vi "Execute Command Script.vi"(7 "Micropulse # In":i32, 8 "error in (no error)":errorcluster, 10 "String in":string) -> (0 "error out":errorcluster, 2 "Transmitted string out":string, 5 "Micropulse # Out":i32)   [LabVIEW 2026, in "MicroPulse_Driver.lvlib"]
doc: "Execute a native Micropulse command (or set of commands separated by carriage returns).\n\n<b>IMPORTANT:</b> Only use this VI if you are familiar with the Micropulse command set and are confident that the commands you are entering are free from errors."
uses:
  MicroPulse_Driver.lvlib
  Private/MP-Registry Action-Enum.ctl
  <vilib>/Utility/error.llb/Trim Whitespace One-Sided.vi
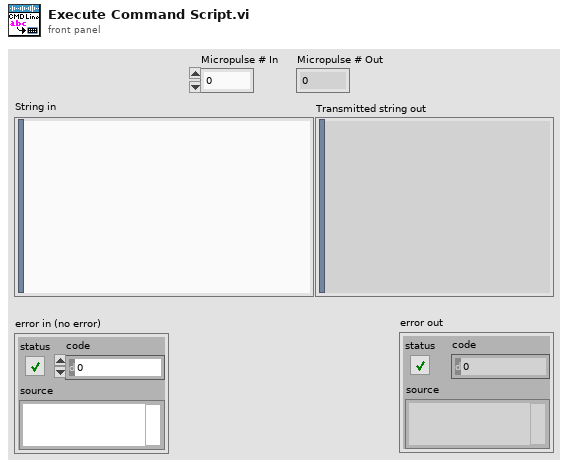
[diagram p1: front panel]
types:
  T1 = typedef "MicroPulse_Driver.lvlib/MP-Registry Action-Enum.ctl" = enum16{"Read", "Add Test", "Add Command", "Add Gate Command", "Add Encoder Command", "Clear Command  List", "Set Registry", "Set System Details", "Set DOF", "Set Velocity", "Disable Asynch Reads", "Enable Asynch Reads", "Add Connection", "Disconnect", "Shutdown"}
  T2 = typedef "Micropulse.lvlib/TCP config.ctl" = cluster{"Connection ID":refnum<k5>, "IP address":string, "host port":u16, "OC timeout":i32, "Read timeout":i32, "Write timeout":i32}
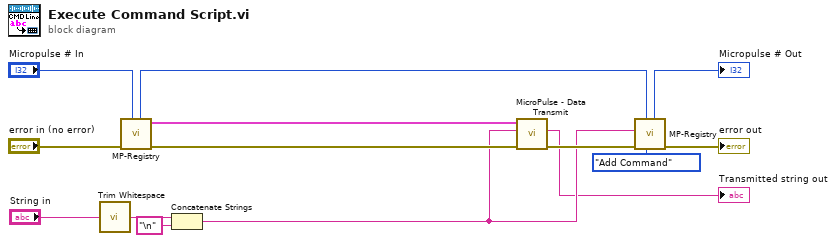
[diagram p0: block diagram]
diagram:
  n1 = call <vilib>:"Trim Whitespace.vi"("string"="String in") -> ("trimmed string"=w4:string)  [unwired: 1 in]
  n2 = call "MP-Registry.vi"("Micropulse # In"="Micropulse # In", "error in (no error)"="error in (no error)") -> ("error out"=w10:errorcluster, "TCP config"=w9:T2, "Micropulse # Out"=w6:i32)  [unwired: 6 in, 1 out]
  n3 = Concatenate Strings(w4, "\n" ("string")) -> (w2:string)
  n4 = call "MicroPulse - Data Transmit.vi"("error in (no error)"=w10, "data"=w2, "TCP config"=w9) -> ("error out"=w7:errorcluster, "status  string"=→"Transmitted string out":string)  [unwired: 6 in, 1 out]
  n5 = call "MP-Registry.vi"("Action"=MP-Registry_Action-Enum."Add Command", "Micropulse # In"=w6, "error in (no error)"=w7, "Data in"=w2) -> ("error out"=→"error out":errorcluster, "Micropulse # Out"=→"Micropulse # Out":i32)  [unwired: 4 in, 2 out]
